vi "ATS_TimeOut_Estimate.vi"(5 "Mult (20)":u32=20, 6 "Rec.Length (B)":u32, 7 "Clock_Value":dbl format="%.2p") -> (3 "TimeOut":dbl format="%.2p")   [LabVIEW 2015]
doc: "_____AlazarTech, Scope_____\n\nEvaluate the Ideal TimeOut in Auto mode."
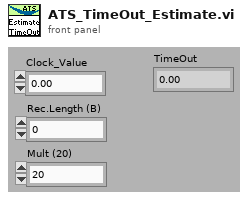
[diagram p1: front panel]
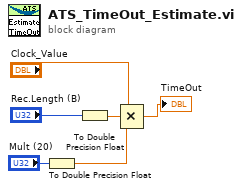
[diagram p0: block diagram]
diagram:
  n1 = To Double Precision Float(number="Mult (20)") -> (double precision float=w4:dbl)
  n2 = To Double Precision Float(number="Rec.Length (B)") -> (double precision float=w1:dbl)
  n3 = Compound Arithmetic op=MULTIPLY("Clock_Value", w1, w4) -> (→"TimeOut":dbl)
